vi "RTD or Thermistor - Continuous Input.vi"() -> ()   [LabVIEW 2022 SP3]
doc: "This example demonstrates how to continuously acquire buffered RTD or Thermistor measurements using a DAQmx device.\n\nFor instructions on how to connect your signals to the DAQ device, refer to your device documentation."
uses:
  <vilib>/Utility/error.llb/DialogType.ctl
  <vilib>/DAQmx/read.llb/DAQmx Read (Analog 1D Wfm NChan NSamp).vi
  <vilib>/DAQmx/create/channels.llb/DAQmx Create Channel (AI-Temperature-RTD).vi
  <vilib>/DAQmx/create/channels.llb/DAQmx Create Channel (AI-Temperature-Thermistor-Iex).vi
  <vilib>/DAQmx/configure/timing.llb/DAQmx Timing (Sample Clock).vi
  <vilib>/DAQmx/configure/task.llb/DAQmx Configure Logging (TDMS).vi
  <vilib>/DAQmx/configure/trigger.llb/DAQmx Start Trigger (Digital Edge).vi
  <vilib>/DAQmx/configure/trigger.llb/DAQmx Start Trigger (Time).vi
  <vilib>/DAQmx/configure/trigger.llb/DAQmx Start Trigger (Analog Edge).vi
  <vilib>/DAQmx/miscellaneous.llb/DAQmx Fill In Error Info.vi
  <resource>/objmgr/daqmx.rc
panel:
  in  "Trigger Type":T1(tab)
  in  "Digital Start Trigger Edge":i32(ring)=10280 caption="Edge" items=["Rising"=10280, "Falling"=10171]
  in  "Digital Start Trigger Source":tag="/Dev1/PFI0" caption="Source"
  in  "Digital Pause Trigger Pause When":i32(ring)=10192 caption="Pause When" items=["High"=10192, "Low"=10214]
  in  "Digital Pause Trigger Source":tag="/Dev1/PFI0" caption="Source"
  in  "Analog Start Trigger Level":dbl caption="Level" format="%0.2f"
  in  "Analog Start Trigger Hysteresis":dbl caption="Hysteresis" format="%.2f"
  in  "Analog Start Trigger Slope":i32(ring)=10280 caption="Slope" items=["Rising"=10280, "Falling"=10171]
  in  "Analog Start Trigger Source":string="APFI0" caption="Source"
  in  "Analog Pause Trigger Source":string="APFI0" caption="Source"
  in  "Analog Pause Trigger Pause When":i32(ring)=10093 caption="Pause When" items=["Above Level"=10093, "Below Level"=10107]
  in  "Analog Pause Trigger Level":dbl caption="Level" format="%.2f"
  in  "When":timestamp
  in  "Select Time\nManually":bool
  in  "TDMS File Path":path
  in  "Logging Mode":i32(ring)=10231 items=["Off"=10231, "Log and Read"=15842]
  in  "Sample Clock Source":tag="OnboardClock"
  in  "Samples per Loop":i32=100
  in  "Current Excitation Source":i32(ring)=10167 items=["Internal"=10200, "External"=10167, "None"=10230]
  in  "Resistance Configuration":i32(ring)=4 items=["2-Wire"=2, "3-Wire"=3, "4-Wire"=4]
  out "Actual Sample Rate (Hz)":dbl
  in  "Tab Control":enum32{"RTD", "Thermistor"}(tab)
  in  "RTD Parameters":T2={"Sensor Resistance at 0 deg C"=100.0, "RTD Type"=12481} {"RTD Type" items=["Pt3750"=12481, "Pt3851"=10071, "Pt3911"=12482, "Pt3916"=10069, "Pt3920"=10053, "Pt3928"=12483, "Custom"=10137]; "Sensor Resistance at 0 deg C" format="%1_5g"}
  in  "Thermistor Parameters":cluster{"A":dbl, "B":dbl, "C":dbl}={"A"=0.001295361, "B"=0.0002343159, "C"=1.018703e-07} {"C" format="%^0.5e"; "B" format="%^0.5e"; "A" format="%^0.5e"}
  in  "Stop":bool
  in  "Sample Rate (Hz)":dbl=1000.0 format="%0.2f"
  out "Waveform Chart":waveform(dbl)[](graph)
  in  "Minimum Value (deg C)":dbl format="%0.2f"
  in  "Maximum Value (deg C)":dbl=100.0 format="%0.2f"
  in  "Physical Channel":tag="Dev1/ai0"
  in  "Current Excitation (A)":dbl=0.0001 format="%0.5f"
  # "Channel Settings"
  # "Acquired Data"
  # "Trigger Settings"
  # "Timing Settings"
  # "Logging Settings"
  # "To enable triggers, select a tab above, and configure the settings.\n\nNot all hardware supports all trigger types. Refer to your device documentation for more information."
  # "This trigger type is not supported in continuous sample timing. \n\nRefer to your device documentation for more information on which triggers are supported."
  # "This trigger type is not supported in continuous sample timing. \n\nRefer to your device documentation for more information on which triggers are supported."
  # "If time is not manually set, task will begin after 10 seconds"
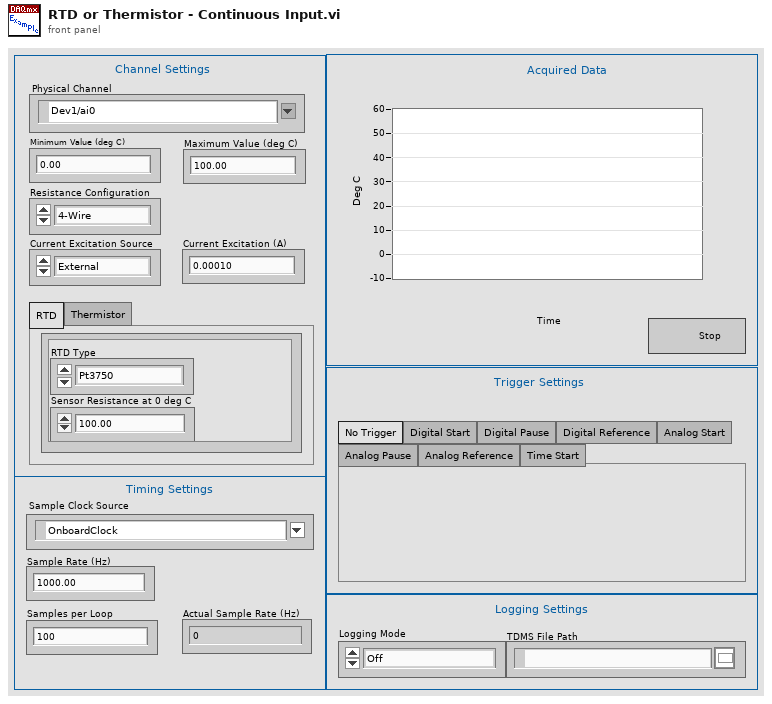
[diagram p1: front panel]
types:
  T1 = enum32{"No Trigger", "Digital Start", "Digital Pause", "Digital Reference", "Analog Start", "Analog Pause", "Analog Reference", "Time Start"}
  T2 = cluster{"Sensor Resistance at 0 deg C":dbl, "RTD Type":i32}
  T3 = typedef "DialogType.ctl" = u16
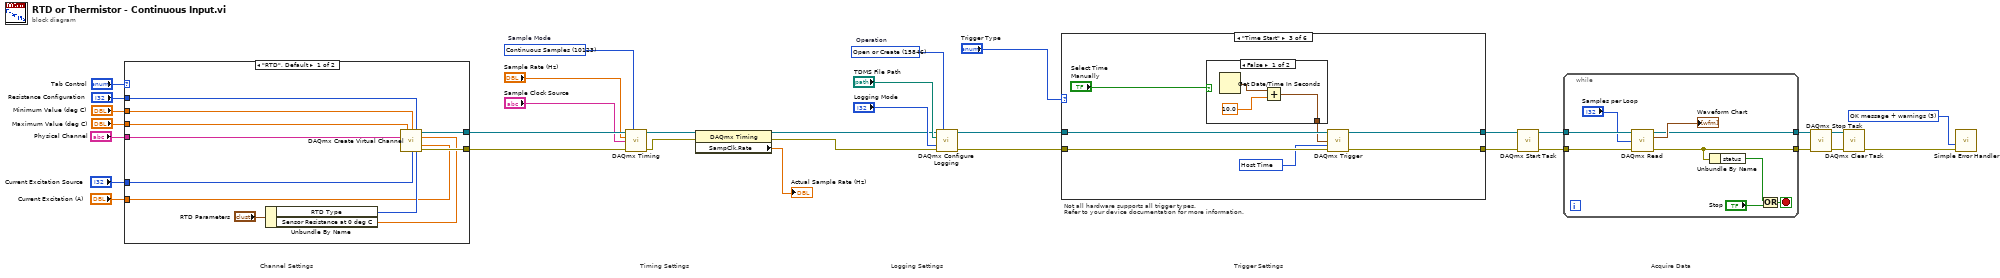
[diagram p0: block diagram]
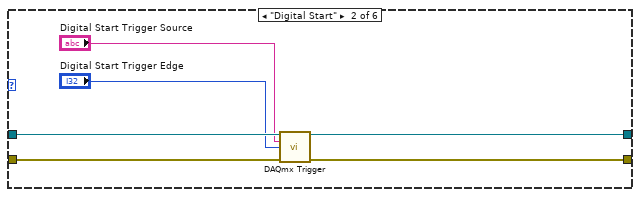
[diagram p3: hidden frame]
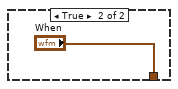
[diagram p4: hidden frame]
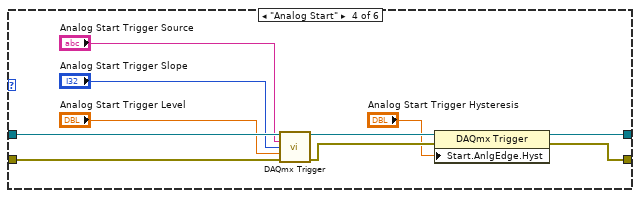
[diagram p5: hidden frame]
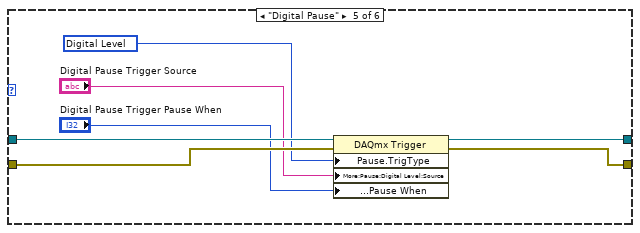
[diagram p6: hidden frame]
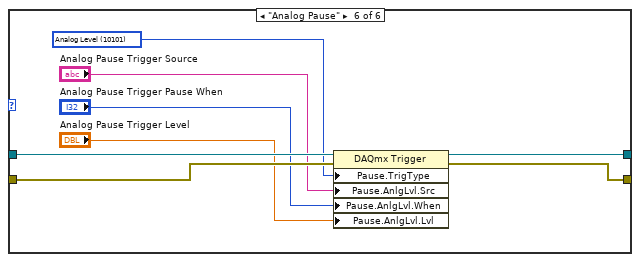
[diagram p7: hidden frame]
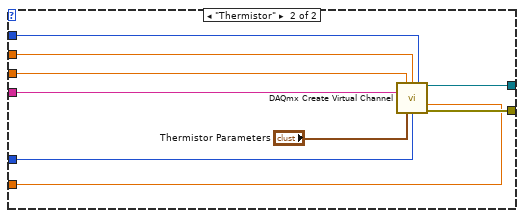
[diagram p8: hidden frame]
diagram:
  w11 = 15846 items=["Open"=10437, "Open or Create"=15846, "Create or Replace"=15847, "Create"=15848]  # Operation
  w31 = 10123 items=["Finite Samples"=10178, "Continuous Samples"=10123, "Hardware Timed Single Point"=12522]  # Sample Mode
  w18 = T3 3 items=["no dialog", "OK message", "continue or stop message", "OK message + warnings", "continue/stop + warnings"] ("Type of Dialog")
  # "Trigger Settings"
  # "Not all hardware supports all trigger types.\nRefer to your device documentation for more information."
  # "Logging Settings"
  # "Acquire Data"
  # "Timing Settings"
  # "Channel Settings"
  n1 = case shown="\"RTD\", Default" "Tab Control" {
    tunnel: [w41 w52] -> w33
    tunnel: [w40 w51] -> w23
    tunnel: "Minimum Value (deg C)" -> [w44 w50]
    tunnel: "Maximum Value (deg C)" -> [w43 w49]
    tunnel: "Physical Channel" -> [w37 w48]
    tunnel: "Resistance Configuration" -> [w42 w47]
    tunnel: "Current Excitation (A)" -> [w35 w46]
    tunnel: "Current Excitation Source" -> [w34 w45]
    frame "RTD", Default {
      n2 = Unbundle By Name("RTD Parameters") -> ("RTD Type"=w36:i32, "Sensor Resistance at 0 deg C"=w38:dbl)
      n3 = call-poly <vilib>:"DAQmx Create Virtual Channel.vi"("maximum value"=w43, "minimum value"=w44, "resistance configuration"=w42, "physical channels"=w37, "r0"=w38, "current excitation value"=w35, "current excitation source"=w34, "rtd type"=w36) -> ("task out"=w41:refnum<k21>, "error out"=w40:errorcluster)  [unwired: 6 in]
    }
    frame "Thermistor" {
      n4 = call-poly <vilib>:"DAQmx Create Virtual Channel.vi"("maximum value"=w49, "minimum value"=w50, "resistance configuration"=w47, "physical channels"=w48, "current excitation value"=w46, "thermistor characteristics"="Thermistor Parameters", "current excitation source"=w45) -> ("task out"=w52:refnum<k21>, "error out"=w51:errorcluster)  [unwired: 7 in]
    }
  }
  n5 = call-poly <vilib>:"DAQmx Timing.vi"("task/channels in"=w33, "sample mode"=w31, "rate"="Sample Rate (Hz)", "source"="Sample Clock Source", "error in"=w23) -> ("task out"=w22:refnum<k21>, "error out"=w21:errorcluster)  [unwired: 9 in]
  n6 = property class="DAQmx Timing"(reference=w22, error in=w21) -> (reference out=w7:refnum<k21>, error out=w6:errorcluster, "SampClk.Rate"=→"Actual Sample Rate (Hz)":dbl)
  n7 = call-poly <vilib>:"DAQmx Configure Logging.vi"("task/channels in"=w7, "operation"=w11, "file path"="TDMS File Path", "logging mode"="Logging Mode", "error in"=w6) -> ("task out"=w1:refnum<k21>, "error out"=w2:errorcluster)  [unwired: 9 in]
  n8 = case shown="\"Time Start\"" "Trigger Type" {
    tunnel: w1 -> [w55 w61 w68 w82 w89 w97]
    tunnel: w2 -> [w54 w60 w67 w81 w86 w94]
    tunnel: [w55 w59 w66 w79 w88 w96] -> w4
    tunnel: [w54 w58 w65 w78 w87 w95] -> w3
    frame "No Trigger", Default {
    }
    frame "Digital Start" {
      n9 = call-poly <vilib>:"DAQmx Trigger.vi"("task/channels in"=w61, "source"="Digital Start Trigger Source", "edge"="Digital Start Trigger Edge", "error in"=w60) -> ("task out"=w59:refnum<k21>, "error out"=w58:errorcluster)  [unwired: 10 in]
    }
    frame "Time Start" {
      w64 = 16126 items=["Host Time"=16126, "I/O Device Time"=16127] ("timescale")
      n10 = case shown="False" "Select Time\nManually" {
        tunnel: [w71 "When"] -> w62
        frame False {
          n11 = Get Date/Time In Seconds() -> (seconds since 1Jan1904=w70:timestamp)
          n12 = Add(x=w70, y=10.0) -> (x+y=w71:timestamp)
        }
        frame True {
        }
      }
      n13 = call-poly <vilib>:"DAQmx Trigger.vi"("task/channels in"=w68, "when"=w62, "timescale"=w64, "error in"=w67) -> ("task out"=w66:refnum<k21>, "error out"=w65:errorcluster)  [unwired: 10 in]
    }
    frame "Analog Start" {
      n14 = call-poly <vilib>:"DAQmx Trigger.vi"("task/channels in"=w82, "source"="Analog Start Trigger Source", "slope"="Analog Start Trigger Slope", "level"="Analog Start Trigger Level", "error in"=w81) -> ("task out"=w77:refnum<k21>, "error out"=w76:errorcluster)  [unwired: 9 in]
      n15 = property class="DAQmx Trigger"(reference=w77, error in=w76, "Start.AnlgEdge.Hyst"="Analog Start Trigger Hysteresis") -> (reference out=w79:refnum<k21>, error out=w78:errorcluster)
    }
    frame "Digital Pause" {
      w85 = 10152 items=["Analog Level"=10101, "Analog Window"=10103, "Digital Level"=10152, "Digital Pattern"=10398, "None"=10230] ("Pause.TrigType")
      n16 = property class="DAQmx Trigger"(reference=w89, error in=w86, "Pause.TrigType"=w85, "More:Pause:Digital Level:Source"="Digital Pause Trigger Source", "More:Pause:Digital Level:Pause When"="Digital Pause Trigger Pause When") -> (reference out=w88:refnum<k21>, error out=w87:errorcluster)
    }
    frame "Analog Pause" {
      w93 = 10101 items=["Analog Level"=10101, "Analog Window"=10103, "Digital Level"=10152, "Digital Pattern"=10398, "None"=10230] ("Pause.TrigType")
      n17 = property class="DAQmx Trigger"(reference=w97, error in=w94, "Pause.TrigType"=w93, "Pause.AnlgLvl.Src"="Analog Pause Trigger Source", "Pause.AnlgLvl.When"="Analog Pause Trigger Pause When", "Pause.AnlgLvl.Lvl"="Analog Pause Trigger Level") -> (reference out=w96:refnum<k21>, error out=w95:errorcluster)
    }
  }
  n18 = call <vilib>:"DAQmx Start Task.vi"("task/channels in"=w4, "error in"=w3) -> ("task out"=w24:refnum<k21>, "error out"=w25:errorcluster)  [unwired: 12 in]
  n19 = while {
    tunnel: w24 -> [w106]
    tunnel: w25 -> [w105]
    tunnel: [w102] -> w14
    tunnel: [w103] -> w15
    stop <- w100 stop-if-true
    n20 = call-poly <vilib>:"DAQmx Read.vi"("task/channels in"=w106, "number of samples per channel"="Samples per Loop", "error in"=w105) -> ("task out"=w103:refnum<k21>, "data"=→"Waveform Chart":waveform(dbl)[], "error out"=w102:errorcluster)  [unwired: 10 in]
    n21 = Unbundle By Name(w102) -> ("status"=w101:bool)
    n22 = Or(x=w101, y="Stop") -> (x .or. y?=w100:bool)
  }
  n23 = call <vilib>:"DAQmx Stop Task.vi"("task/channels in"=w15, "error in"=w14) -> ("task out"=w13:refnum<k21>, "error out"=w12:errorcluster)  [unwired: 12 in]
  n24 = call <vilib>:"DAQmx Clear Task.vi"("task in"=w13, "error in"=w12) -> ("error out"=w19:errorcluster)  [unwired: 13 in]
  n25 = call <vilib>:"Simple Error Handler.vi"("type of dialog (OK msg:1)"=w18, "error in (no error)"=w19) -> ()  [unwired: 3 in, 5 out]
